vi "TestCamA.vi"() -> ()   [LabVIEW 2018]
uses:
  <vilib>/vision/driver/NI_Vision_Acquisition_Software.lvlib
  <vilib>/myRIO/Instrument Drivers/Onboard IO/PWM/typedefs/PWM Configuration.ctl
  <vilib>/myRIO/Instrument Drivers/Onboard IO/PWM/PWM.lvlib
  <vilib>/myRIO/Common/Instrument Driver Framework/myRIO v1.0/PWM/typedefs/PWM Channels Enum.ctl
  <vilib>/myRIO/Common/Instrument Driver Framework/Utilities/typedefs/Generic FPGA Reference.ctl
  <vilib>/myRIO/Common/Instrument Driver Framework/Utilities/typedefs/myRIO v1.0 Reference.ctl
  <vilib>/myRIO/Common/Instrument Driver Framework/Utilities/typedefs/Hardware Version Enum.ctl
  <vilib>/myRIO/Common/Instrument Driver Framework/Utilities/typedefs/myRIO Generic Hardware Reference.ctl
  <vilib>/myRIO/Instrument Drivers/Onboard IO/PWM/typedefs/PWM Reference.ctl
  <vilib>/myRIO/Instrument Drivers/Onboard IO/PWM/vis/Set Duty Cycle and Frequency.vi
  <vilib>/userdefined/High Color/nirio_resource_hc.ctl
  <vilib>/myRIO/Common/Instrument Driver Framework/myRIO v1.0/PWM/vis/myRIO v1.1 Open PWM.vi
  <vilib>/myRIO/Instrument Drivers/Onboard IO/PWM/vis/myRIO PWM Open.xnode
  <vilib>/myRIO/Common/Instrument Driver Framework/Utilities/vis/Is FPGA Ref Available.vi
  <vilib>/myRIO/Express VI/Onboard IO/PWM/PWM Express VI.xnode
  <vilib>/myRIO/Common/Instrument Driver Framework/myRIO v1.0/DIO/typedefs/DIO Channels Enum.ctl
  <vilib>/myRIO/Common/Instrument Driver Framework/myRIO v1.0/DIO/typedefs/DIO Channels List.ctl
  <vilib>/myRIO/Instrument Drivers/Onboard IO/DIO/typedefs/DIO Reference.ctl
  <vilib>/myRIO/Instrument Drivers/Onboard IO/DIO/DIO.lvlib
  <vilib>/myRIO/Instrument Drivers/Onboard IO/DIO/vis/Write.vi
  <vilib>/myRIO/Common/Instrument Driver Framework/myRIO v1.0/DIO/vis/myRIO v1.1 Open DIO.vi
  <vilib>/myRIO/Instrument Drivers/Onboard IO/DIO/vis/myRIO DIO Open.xnode
  <vilib>/myRIO/Express VI/Onboard IO/DO/DO Express VI.xnode
  <vilib>/myRIO/Instrument Drivers/Utilities/Utilities.lvlib
  <vilib>/userdefined/High Color/IMAQdx.ctl
panel:
  in  "Load Image":bool
  in  "Select Image":string(combo)="AA"
  out "Image Load":T1(plugin-control)
  in  "File Path":path=path "c:/AA.png"
  in  "Save Image":bool
  in  "QR CODE":bool
  out "dcolor":i32
  out "ucolor":i32
  out "QR_CODE":string
  in  "Duty Cycle":dbl=0.6
  in  "ENABLE":bool=TRUE
  out "Image":T1(plugin-control)
  in  "stop":bool
  out "error out":errorcluster
  in  "Session In":T2="cam1"
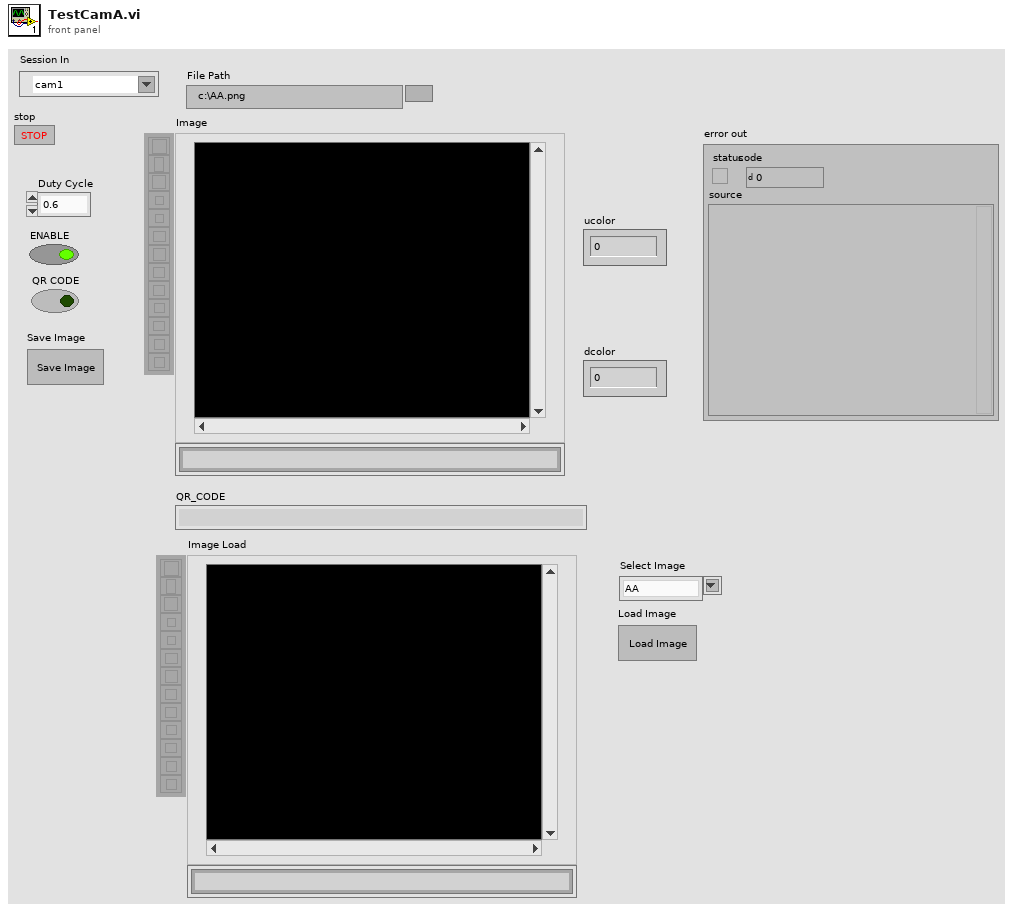
[diagram p1: front panel]
types:
  T1 = typedef "IMAQ Image.ctl" = refnum<image>
  T2 = typedef "IMAQdx.ctl" = refnum<k21>
  T3 = cluster{"proportional gain (Kc)":dbl, "integral time (Ti, min)":dbl, "derivative time (Td, min)":dbl}
  T4 = typedef "PWM.lvlib/PWM Reference.ctl" = cluster{"myRIO Reference":T5, "PWM Channels Enum":T9, "PWM Configuration":T10}
  T5 = typedef "myRIO Generic Hardware Reference.ctl" = cluster{"myRIO Model":T6, "myRIO Hardware Reference":T7}
  T6 = typedef "Hardware Version Enum.ctl" = enum16{"Unknown", "myRIO-1900", "myRIO-1950", "roboRIO", "NI ELVIS RIO CM", "ELVIS III"}
  T7 = typedef "myRIO v1.0 Reference.ctl" = cluster{"Generic FPGA Reference":T8, "Allow multiple opens":bool}
  T8 = typedef "Generic FPGA Reference.ctl" = refnum<k20>
  T9 = typedef "PWM Channels Enum.ctl" = enum16{"Not Connected", "C/PWM0", "C/PWM1", "A/PWM0", "A/PWM1", "A/PWM2", "A/PWM3", "A/PWM4", "A/PWM5", "A/PWM6", "A/PWM7", "A/PWM8", "A/PWM9", "A/PWM10", "A/PWM11", "A/PWM12", "A/PWM13", "A/PWM14", "A/PWM15", "A/PWM16", "A/PWM17", "A/PWM18", "A/PWM19", "B/PWM0", "B/PWM1", "B/PWM2", "B/PWM3", "B/PWM4", "B/PWM5", "B/PWM6", "B/PWM7", "B/PWM8", "B/PWM9", "B/PWM10", "B/PWM11", "B/PWM12", "B/PWM13", "B/PWM14", "B/PWM15", "B/PWM16", "B/PWM17", "B/PWM18", "B/PWM19", "PWM/PWM0", "PWM/PWM1", "PWM/PWM2", "PWM/PWM3", "PWM/PWM4", "PWM/PWM5", "PWM/PWM6", "PWM/PWM7", "PWM/PWM8", "PWM/PWM9"}
  T10 = typedef "PWM.lvlib/PWM Configuration.ctl" = cluster{"Frequency":dbl, "Duty Cycle":dbl}
  T11 = typedef "nirio_resource_hc.ctl" = tag
  T12 = typedef "DIO.lvlib/DIO Reference.ctl" = cluster{"myRIO Reference":T5, "DIO Channels List":T13}
  T13 = typedef "DIO Channels List.ctl" = T14[]
  T14 = typedef "DIO Channels Enum.ctl" = enum16{"Not Connected", "C/DIO0", "C/DIO1", "C/DIO2", "C/DIO3", "C/DIO4", "C/DIO5", "C/DIO6", "C/DIO7", "A/DIO0", "A/DIO1", "A/DIO2", "A/DIO3", "A/DIO4", "A/DIO5", "A/DIO6", "A/DIO7", "A/DIO8", "A/DIO9", "A/DIO10", "A/DIO11", "A/DIO12", "A/DIO13", "A/DIO14", "A/DIO15", "A/DIO16", "A/DIO17", "A/DIO18", "A/DIO19", "B/DIO0", "B/DIO1", "B/DIO2", "B/DIO3", "B/DIO4", "B/DIO5", "B/DIO6", "B/DIO7", "B/DIO8", "B/DIO9", "B/DIO10", "B/DIO11", "B/DIO12", "B/DIO13", "B/DIO14", "B/DIO15", "B/DIO16", "B/DIO17", "B/DIO18", "B/DIO19", "LED0", "LED1", "LED2", "LED3", "Button0", "DIO/DIO0", "DIO/DIO1", "DIO/DIO2", "DIO/DIO3", "DIO/DIO4", "DIO/DIO5", "DIO/DIO6", "DIO/DIO7", "DIO/DIO8", "DIO/DIO9", "SPI/CS0", "SPI/CS1", "SPI/CS2", "SPI/CS3", "LED RADIO (Green)", "LED RADIO (Red)", "LED COMM (Green)", "LED COMM (Red)", "LED MODE (Green)", "LED MODE (Red)"}
  T15 = cluster{"Speed A(mm/s)":dbl, "Speed B(mm/s)":dbl, "Speed C(mm/s)":dbl}
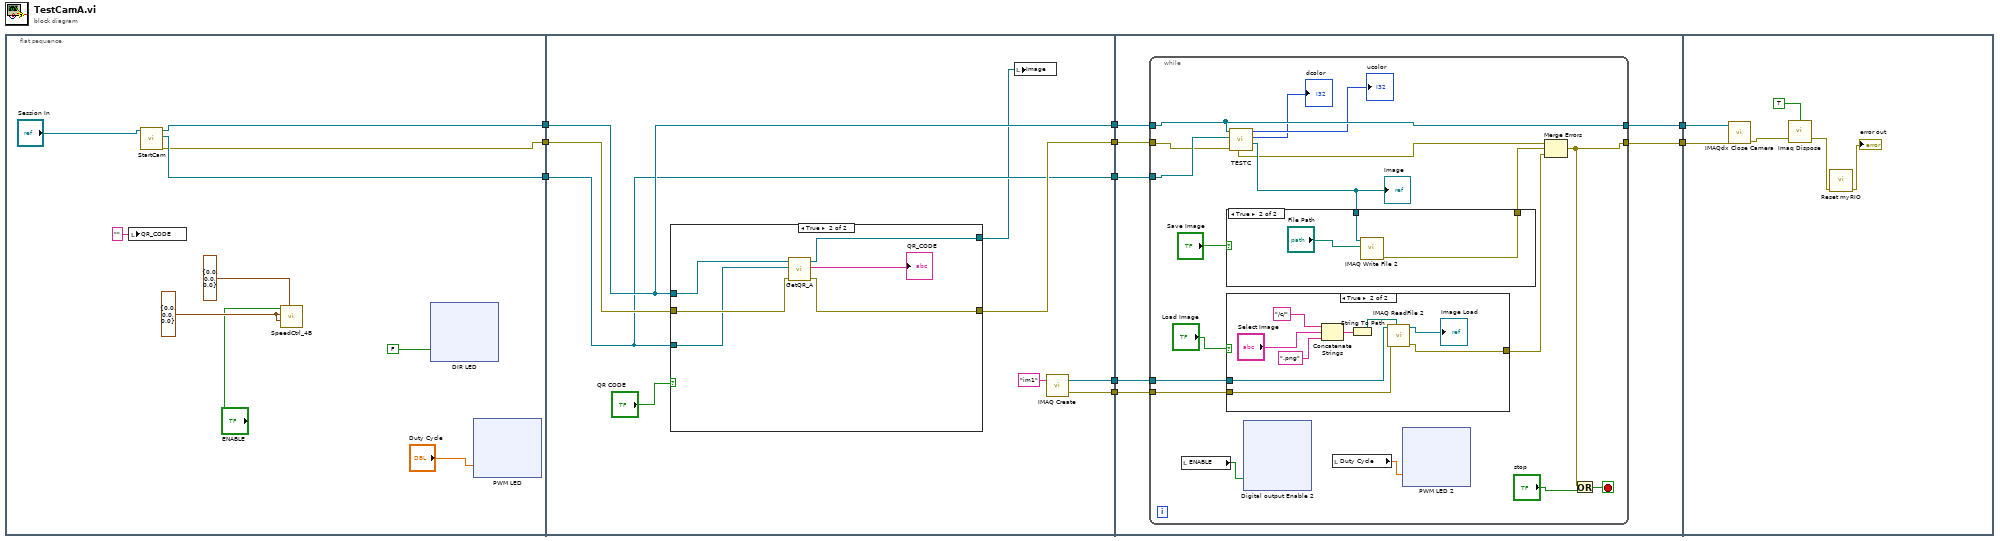
[diagram p0: block diagram]
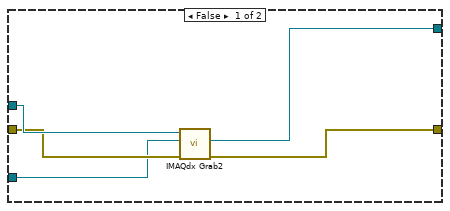
[diagram p2: hidden frame]
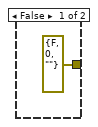
[diagram p3: hidden frame]
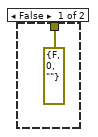
[diagram p4: hidden frame]
diagram:
  n1 = flat-sequence {
    tunnel: [w18] -> w8
    tunnel: [w16] -> w6
    tunnel: [w17] -> w4
    tunnel: w8 -> [w99]
    tunnel: [w99] -> w7
    tunnel: w6 -> [w98]
    tunnel: [w97] -> w5
    tunnel: w4 -> [w96]
    tunnel: [w96] -> w3
    tunnel: [w92] -> w2
    tunnel: [w91] -> w1
    tunnel: w7 -> [w117]
    tunnel: [w116] -> w10
    tunnel: w5 -> [w115]
    tunnel: [w114] -> w9
    tunnel: w3 -> [w113]
    tunnel: w2 -> [w112]
    tunnel: w1 -> [w111]
    tunnel: w10 -> [w225]
    tunnel: w9 -> [w224]
    frame #0 {
      w13 = T15 {"Speed A(mm/s)"=0.0, "Speed B(mm/s)"=0.0, "Speed C(mm/s)"=0.0} ("Speed Now")
      n2 = local write "QR_CODE"("" ("QR_CODE")) -> ()
      n3 = call "StartCam.vi"("Session In"="Session In") -> ("error out"=w16:errorcluster, "New Image"=w17:T1, "Session Out"=w18:T2)  [unwired: 8 in]
      n4 = call "SpeedCtrl_4B.vi"("PID gains"=T3 {"proportional gain (Kc)"=0.0, "integral time (Ti, min)"=0.0, "derivative time (Td, min)"=0.0}, "Target Spd. \nmm/s"=w13, "Speed Now"=w13, "Enable"="ENABLE") -> ()  [unwired: 7 in, 1 out]
      n5 = xnode "DIR LED"("DIRC (C/DIO5 (DIO5))"=FALSE) -> ()  [unwired: 1 in, 1 out]
      n6 = xnode "PWM LED"("Duty Cycle"="Duty Cycle") -> ()  [unwired: 1 in, 1 out]
    }
    frame #1 {
      n7 = case shown="True" "QR CODE" {
        tunnel: w99 -> [w104 w110]
        tunnel: w98 -> [w103 w108]
        tunnel: [w100 w107] -> w97
        tunnel: w96 -> [w102 w106]
        tunnel: [w101 w105] -> w95
        frame False {
          n8 = call <vilib>:"IMAQdx Grab2.vi"("error in"=w103, "Image In"=w102, "Session In"=w104) -> ("error out"=w100:errorcluster, "Image Out"=w101:T1)  [unwired: 5 in, 2 out]
        }
        frame True {
          n9 = call "GetQR_A.vi"("error in"=w108, "Image In"=w106, "Session In"=w110) -> ("error out"=w107:errorcluster, "QR_CODE"=→"QR_CODE":string, "Image Out"=w105:T1)  [unwired: 5 in, 1 out]
        }
      }
      n10 = local write "Image"(w95) -> ()
      n11 = call "IMAQ Create"("Image Name"="im1") -> ("New Image"=w92:T1, "error out"=w91:errorcluster)  [unwired: 4 in]
    }
    frame #2 {
      n12 = while {
        tunnel: w113 -> [w135]
        tunnel: w117 -> [w133]
        tunnel: [w133] -> w116
        tunnel: w115 -> [w134]
        tunnel: [w124] -> w114
        tunnel: w112 -> [w119]
        tunnel: w111 -> [w118]
        stop <- w126 stop-if-true
        n13 = local read "ENABLE"() -> (w121:bool)
        n14 = case shown="True" "Load Image" {
          tunnel: [errorcluster {"status"=FALSE, "code"=0, "source"=""} ("error out") w209] -> w123
          tunnel: w119 -> [_ w208]
          tunnel: w118 -> [_ w207]
          frame False {
          }
          frame True {
            n15 = Concatenate Strings("/c/" ("string"), "Select Image", ".png" ("string")) -> (w212:string)
            n16 = String To Path(string=w212) -> (path=w211:path)
            n17 = call "IMAQ ReadFile 2"("File Path"=w211, "error in (no error)"=w207, "Image"=w208) -> ("error out"=w209:errorcluster, "Image Out"=→"Image Load":T1)  [unwired: 4 in, 3 out]
          }
        }
        n18 = call "TESTC.vi"("error in"=w134, "Image In"=w135, "Session In"=w133) -> ("Image Out"=w129:T1, "dcolor"=→"dcolor":i32, "ucolor"=→"ucolor":i32, "error out"=w128:errorcluster)  [unwired: 2 in, 3 out]
        "Image" <- w129
        n19 = case shown="True" "Save Image" {
          tunnel: w129 -> [_ w219]
          tunnel: [errorcluster {"status"=FALSE, "code"=0, "source"=""} ("error out") w218] -> w127
          frame False {
          }
          frame True {
            n20 = call-poly "IMAQ Write File 2"("File Path"="File Path", "Image"=w219) -> ("error out"=w218:errorcluster)  [unwired: 8 in, 1 out]
          }
        }
        n21 = xnode "Digital output Enable 2"("ENABLE (A/DIO4 (Pin 19))"=w121) -> ()  [unwired: 1 in, 1 out]
        n22 = local read "Duty Cycle"() -> (w120:dbl)
        n23 = xnode "PWM LED 2"("Duty Cycle"=w120) -> ()  [unwired: 1 in, 1 out]
        n24 = Merge Errors(w128, w127, w123) -> (w124:errorcluster)
        n25 = Or(x=w124, y="stop") -> (x .or. y?=w126:bool)
      }
    }
    frame #3 {
      n26 = call <vilib>:"IMAQdx Close Camera.vi"("error in"=w224, "Session In"=w225) -> ("error out"=w223:errorcluster)  [unwired: 9 in]
      n27 = call "Imaq Dispose"("All Images? (No)"=TRUE, "error in (no error)"=w223) -> ("error out"=w221:errorcluster)  [unwired: 4 in]
      n28 = call <vilib>:"Reset myRIO.vi"("error in (no error)"=w221) -> ("error out"=→"error out":errorcluster)  [unwired: 10 in]
    }
  }
